vi "Get SMO Port.vi"(8 "error in (no error)":errorcluster, 11 "Inst.Krohn-Hite-7008Instrument in":refnum<class "Inst.Krohn-Hite-7008.lvclass">) -> (0 "error out":errorcluster, 2 "Port":u16, 3 "Inst.Krohn-Hite-7008Instrument out":refnum<class "Inst.Krohn-Hite-7008.lvclass">)   [LabVIEW 2019, in "Inst.KH7008.lvlib" / "Inst.Krohn-Hite-7008.lvclass"]
uses:
  Inst.Krohn-Hite-7008.lvclass
  <userlib>/LevyLab/Instrument Framework/Instrument Types/Amplifier/Instrument.Amplifier.lvclass
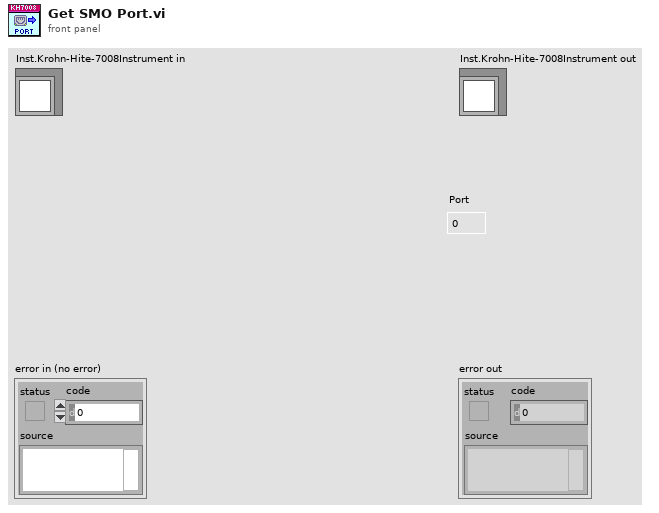
[diagram p1: front panel]
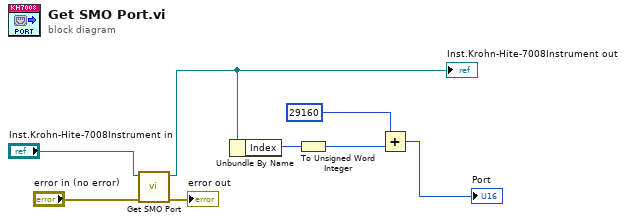
[diagram p0: block diagram]
diagram:
  n1 = call-parent "Get SMO Port.vi"("error in (no error)"="error in (no error)", "Instrument in"="Inst.Krohn-Hite-7008Instrument in") -> ("error out"=→"error out":errorcluster, "Instrument out"=w5:refnum<class "Inst.Krohn-Hite-7008.lvclass">)  [unwired: 7 in, 1 out]
  "Inst.Krohn-Hite-7008Instrument out" <- w5
  n2 = Unbundle By Name(w5) -> ("Index"=w4:i32)
  n3 = To Unsigned Word Integer(number=w4) -> (unsigned 16bit integer=w1:u16)
  n4 = Add(x=u16 29160 ("Port"), y=w1) -> (x+y=→"Port":u16)
